vi "Scale and Ave All Raw Readings.vi"(2 "Scale":dbl[](array[numeric]) format="%.4f", 3 "Offset":dbl[](array[numeric]) format="%.3f", 4 "Input Array":dbl[][](array[numeric]) format="%.2f") -> (0 "Raw Voltage":dbl[](array[numeric]) format="%.3f", 1 "Scaled Array":dbl[](array[numeric]) format="%.3f")   [LabVIEW 2020]
doc: "Takes an array of M by N readings in binary from the A/D board, averages over the N readings and scales to physical units using the calibrations entered. Offset array of M values in volts is added to reading and then multiplied by Scale array of M values.\nScott Hannahs, NHMFL-FSU, July 2021\n<sth@magnet.fsu.edu>"
uses:
  <vilib>/Analysis/baseanly.llb/Mean (DBL).vi
  <vilib>/Analysis/NI_AALBase.lvlib
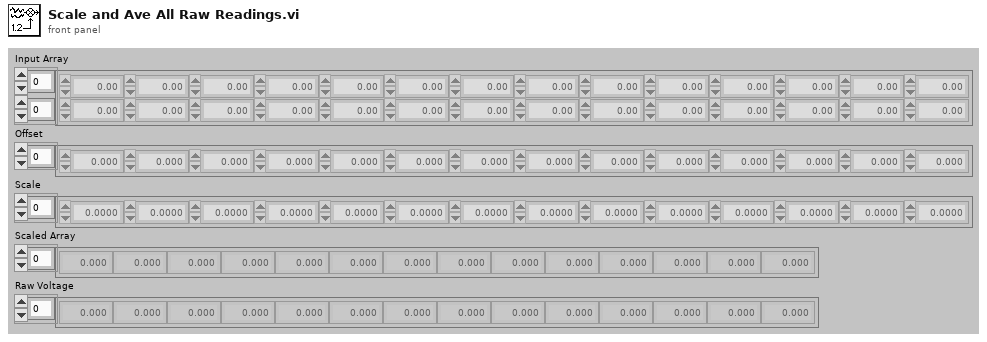
[diagram p1: front panel]
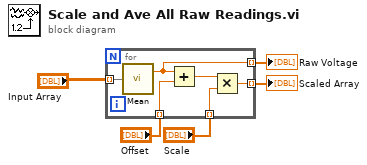
[diagram p0: block diagram]
diagram:
  n1 = for {
    tunnel: [w11] -> w3 mode=indexing
    tunnel: "Offset" -> [w10] mode=indexing
    tunnel: "Scale" -> [w8] mode=indexing
    tunnel: "Input Array" -> [w7] mode=indexing
    tunnel: [w6] -> w1 mode=indexing
    n2 = call-poly <vilib>:"Mean.vi"("X"=w7) -> ("mean"=w6:dbl)  [unwired: 1 out]
    n3 = Add(x=w6, y=w10) -> (x+y=w9:dbl)
    n4 = Multiply(x=w9, y=w8) -> (x*y=w11:dbl)
  }
  "Scaled Array" <- w3
  "Raw Voltage" <- w1
